vi "LVClass_SlopesPostProcessList AddProcessor_DoublePassage.vi"(0 "SlopesPostProcessorList in":refnum<class "SlopesPostProcessorList.lvclass">, 5 "Position":i32, 7 "doublePath":T1, 11 "error in (no error)":errorcluster) -> (4 "SlopesPostProcessorList out":refnum<class "SlopesPostProcessorList.lvclass">, 15 "error out":errorcluster)   [LabVIEW 2020, in "SlopesPostProcessorList.lvclass"]
doc: "Insert a DoublePath processor.\n\n--------------------------------------------------------------------------------\n\n<B>SlopesPostProcessorListIn </B> : SlopesPostProcessorList object.\n<B>SlopesPostProcessorListOut </B> : SlopesPostProcessorList object.\n<B>position </B> : Position of the processor in the SlopesPostProcessorList.\n<B>is_doublePath_active_on_tilt</B> : Is Double path active on tilt.\n<B>is_doublePath_active_on_curv</B> : Is Double path is active on curvature.\n<B>ErrorIn </B> : Error\n<B>ErrorOut </B> : Error\n\n--------------------------------------------------------------------------------"
uses:
  SlopesPostProcessorList.lvclass
  SlopesPostProcessorList - Double passage.ctl
  SlopesPostProcessorList.lvclass/SlopesPostProcessorList.ctl
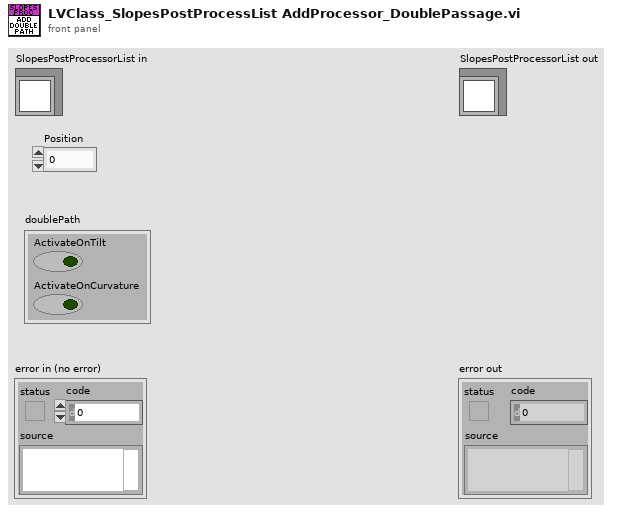
[diagram p1: front panel]
types:
  T1 = typedef "SlopesPostProcessorList - Double passage.ctl" = cluster{"ActivateOnTilt":bool, "ActivateOnCurvature":bool}
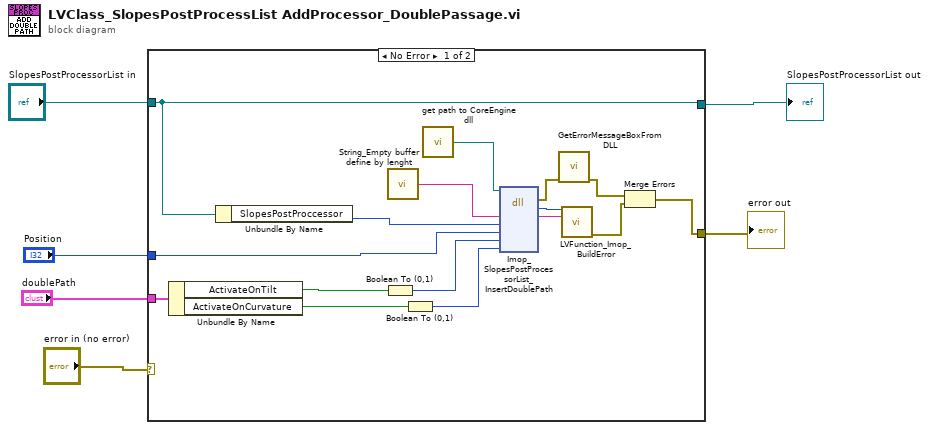
[diagram p0: block diagram]
diagram:
  n1 = case shown="No Error" "error in (no error)" {
    selector: "error in (no error)" -> [_ w23]
    tunnel: "SlopesPostProcessorList in" -> [w15 w24]
    tunnel: [w15 w24] -> w4
    tunnel: [w11 w23] -> w3
    tunnel: "Position" -> [w10 _]
    tunnel: "doublePath" -> [w9 _]
    frame No Error {
      n2 = Unbundle By Name(w9) -> ("ActivateOnTilt"=w8:bool, "ActivateOnCurvature"=w7:bool)
      n3 = Unbundle By Name(w15) -> ("SlopesPostProccessor"=w14:i32)
      n4 = Boolean To (0,1)(Boolean=w8) -> (0, 1=w17:i16)
      n5 = call "String_Empty buffer define by lenght.vi"() -> ("Empty buffer"=w22:string)  [unwired: 1 in]
      n6 = Boolean To (0,1)(Boolean=w7) -> (0, 1=w16:i16)
      n7 = call "get path to CoreEngine dll.vi"() -> ("path to c_interface_vc100.dll"=w19:path)  [unwired: 12 in, 3 out]
      n8 = dll-call lib="D:/soft/HASO_v3/SVN_trunk/ImOpCoreEngine4_LV2011/DLLs/c_interface_vc100.dll" fn="Imop_SlopesPostProcessorList_InsertDoublePath"(path in=w19, "message"=w22, "objet"=w14, "Position"=w10, "double passage activate on tilt"=w17, "double passage activate on curvature"=w16) -> (error out=w18:errorcluster, "return type"=w20:i32, "message"=w21:string)  [unwired: 6 in, 1 out]
      n9 = call "GetErrorMessageBoxFromDLL.vi"("error IN"=w18) -> ("error OUT"=w13:errorcluster)  [unwired: 10 in]
      n10 = call "LVFunction_Imop_BuildError.vi"("code"=w20, "String to Prepend to source (\"\")"=w21) -> ("error out"=w12:errorcluster)  [unwired: 13 in]
      n11 = Merge Errors(w13, w12) -> (w11:errorcluster)
    }
    frame Error {
    }
  }
  "error out" <- w3
  "SlopesPostProcessorList out" <- w4
